vi "server.Add Response (Server Error).vi"(5 "id value":string, 6 "code (-32000 to -32099)":i32=-32000, 7 "jsonrpc":string="2.0", 8 "error in (no error)":errorcluster, 10 "data":refnum<class "JSON Null.lvclass">, 11 "Server in":refnum<class "JSONRPC Server.lvclass">) -> (0 "error out":errorcluster, 1 "response string":string, 3 "Server out":refnum<class "JSONRPC Server.lvclass">)   [LabVIEW 2016, in "JSONRPC Server.lvclass"]
uses:
  JSONRPC Server.lvclass
  <vilib>/NI/JSON Support for LabVIEW/JSON Data Classes/JSON Datatype/JSON Null.lvclass
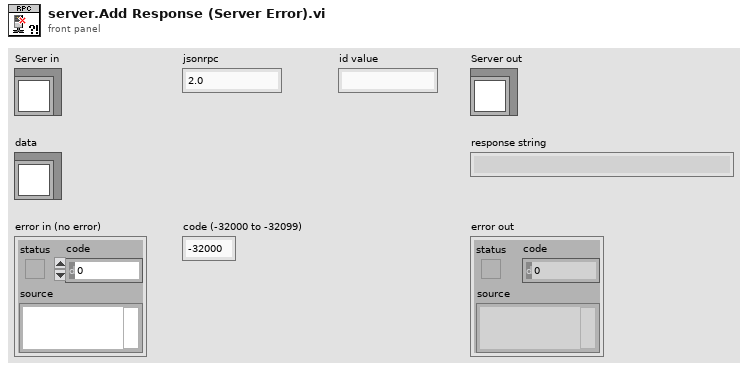
[diagram p1: front panel]
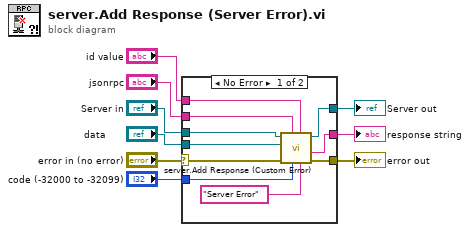
[diagram p0: block diagram]
diagram:
  n1 = case shown="No Error" "error in (no error)" {
    selector: "error in (no error)" -> [w12 w21]
    tunnel: [w13 w21] -> w8
    tunnel: [w18 w20] -> w6
    tunnel: "Server in" -> [w19 w20]
    tunnel: "data" -> [w16 _]
    tunnel: "jsonrpc" -> [w15 _]
    tunnel: "id value" -> [w14 _]
    tunnel: "code (-32000 to -32099)" -> [w11 _]
    tunnel: [w10 _] -> w1
    frame No Error {
      n2 = call "server.Add Response (Custom Error).vi"("message"="Server Error", "id value"=w14, "code"=w11, "jsonrpc"=w15, "error in (no error)"=w12, "data"=w16, "Server in"=w19) -> ("error out"=w13:errorcluster, "response string"=w10:string, "Server out"=w18:refnum<class "JSONRPC Server.lvclass">)  [unwired: 2 in]
    }
    frame Error {
    }
  }
  "error out" <- w8
  "Server out" <- w6
  "response string" <- w1
